vi "PID.vi"(0 "Numeric in":dbl, 1 "P_outer gain":dbl, 2 "Inner PID T/F":bool, 3 "Old (F), new (T) PID":bool, 4 "I_outer gain":dbl, 5 "D_outer gain":dbl, 6 "Velocity (Counts/interval)":i32, 7 "P_inner gain":dbl, 8 "Position (Counts)":i32, 9 "I_inner gain":dbl, 11 "D_inner gain":dbl) -> (14 "Numeric out":dbl)   [LabVIEW 2019]
uses:
  <vilib>/Simulation/Scripting/Companion Diagram/SimConfigNode/SimParams.ctl
  <vilib>/Simulation/Scripting/Companion Diagram/SimConfigNode/_simSolvers.ctl
  <vilib>/Simulation/Implementation/Shared/SIMSCR Execution Mode.ctl
  <vilib>/Simulation/Param Hierarchy/Typedefs/SIMPH Param Control Actions.ctl
  <vilib>/Simulation/Implementation/Shared/NILVSim_ParamChanged.vi
  <vilib>/Simulation/Implementation/Shared/NILVSIM_BeginStep.vi
  <vilib>/Simulation/Implementation/Shared/NILVSim_Manager.vi
  <vilib>/Utility/error.llb/Clear Errors.vi
  <vilib>/Simulation/Implementation/Shared/NILVSim_FinalizeModel.vi
  <vilib>/Simulation/Implementation/Shared/SIM Unbundle Sim Info.vi
  <vilib>/Simulation/Implementation/Shared/NILVSim_Initialize.vi
  <vilib>/Simulation/Utility/Implementation/NILVSim Get Time and IsAcceptedStep.vi
  <vilib>/Simulation/Implementation/Shared/SIMSH Read Queue.vi
  <vilib>/Simulation/Implementation/Shared/NILVSim_GetModelError.vi
  <vilib>/Simulation/Implementation/Shared/SIM Bundle Sim Info.vi
  <vilib>/Simulation/Implementation/XNodeFramework/SimXNode/SimX.xnode
  <vilib>/Simulation/Model Libraries/PID/SIM PID (Parallel).vi
  <vilib>/Simulation/Scripting/Companion Diagram/SimConfigNode/SimDog.xnode
  <vilib>/Simulation/Model Libraries/PID/SIM PID (Academic).vi
  <vilib>/ptbypt/NI_PtbyPt.lvlib
  <vilib>/Simulation/Implementation/Shared/NI_SIM_Implementation.lvlib
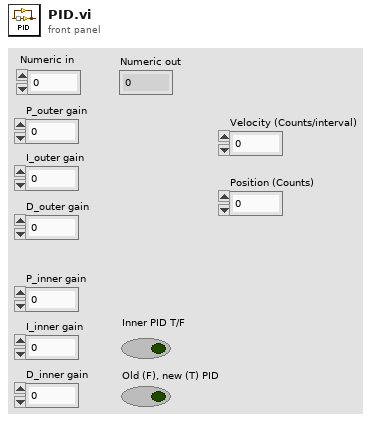
[diagram p1: front panel]
types:
  T1 = enum16{"Simulate to Completion", "Single Time-Step Simulation (Fixed Step Only)"}
  T2 = typedef "SIMSCR Execution Mode.ctl" = enum16{"Simulate to Completion", "Single Time-Step Simulation (Fixed Step Only)"}
  T3 = typedef "SIMPH Param Control Actions.ctl" = enum16{"get params", "set params"}
  T4 = cluster{"SIMSH Sim Time":dbl, "SIM PID Derivative Gain.vi":cluster{"output":dbl}, "SIM PID Derivative Gain.vi - SIMSH":cluster{"SIMSH Sim Time":dbl, "t 3":dbl, "Select 2":cluster{"s? t:f":dbl}, "Equal?":cluster{"x = y?":bool}, "Or":cluster{"x .or. y?":bool}, "Equal To 0?":cluster{"x = 0?":bool}}, "High Frequency [s] (Tf)":dbl, "Gain":cluster{"output":dbl}, "Summation":cluster{"Result":dbl}, "Integral Gain - series.vi":cluster{"output":dbl}, "Integral Gain - series.vi - SIMSH":cluster{"SIMSH Sim Time":dbl, "Select 2":cluster{"s? t:f":dbl}, "integral in gain?":bool, "Integrator":cluster{"output y(t)":dbl}, "Gain 2":cluster{"output":dbl}, "Select":cluster{"s? t:f":dbl}, "Equal To 0?":cluster{"x = 0?":bool}, "Reciprocal":cluster{"1/x":dbl}}}
  T5 = typedef "SimParams.ctl" = cluster{"Initial Time (s)":dbl, "Final Time (s)":dbl, "Step Size (s)":dbl, "ODE Solver":T6, "Minimum Step Size (s)":dbl, "Maximum Step Size (s)":dbl, "Relative Tolerance":dbl, "Absolute Tolerance":dbl, "Software Timing":bool, "Initial Step Size (s)":dbl, "Automatic Fixed Step Size?":bool, "Automatic Discrete Step Size?":bool, "Discrete Step Size (s)":dbl, "Calculate using Time Step":bool, "Solver Wired?":bool, "Prev.Frm.Expected End":u64, "Prev.Frm.Actual End":u64, "Prev.Frm.Finished Late?":bool, "Prev.Iter.Expected End":u64, "Prev.Iter.Actual End":u64, "Prev.Iter.Finished Late?":bool, "Expected Iteration Start":u64, "Actual Iteration Start":u64, "Expected Frame Start":u64, "Actual Frame Start":u64, "Source Name":string, "Name":string, "Period":i64, "Deadline":i64, "Offset":i64, "Start":i64, "Priority":i32, "Timeout":i32, "Processor":i32, "Mode":enum32{"No Change", "Process missed periods, maintain original phase", "Discard missed periods, maintain original phase", "Process missed periods, ignore original phase", "Discard missed periods, ignore original phase"}, "Wakeup reason":enum32{"Normal", "Aborted", "Asynchronous wakeup", "Timing source error", "Timed loop error", "Timeout"}, "Error":errorcluster, "Source Type":string, "Secondary Source Type":string, "Global End Time":u64, "Global Start Time":u64, "Full Solver Reset":bool, "Execution Mode":T2, "Nan/Inf Check":bool, "Custom Solver Library":string, "Solver Is Variable":bool, "custom solver name":string, "Signal Collection Decimation":u32}
  T6 = typedef "_simSolvers.ctl" = enum16{"Runge-Kutta 1 (Euler)", "Runge-Kutta 2", "Runge-Kutta 3", "Runge-Kutta 4", "Runge-Kutta 23 (variable)", "Runge-Kutta 45 (variable)", "BDF (variable)", "Adams-Moulton (variable)", "Rosenbrock (variable)", "Discrete States Only", "SDIRK 4 (variable)", "Radau 5 (variable)", "Radau 9 (variable)", "Radau 13 (variable)", "Radau [Variable Order] (variable)", "Gear's Method (variable)", "Linearizer", "State Query", "Trim Eval", "Custom Solver"}
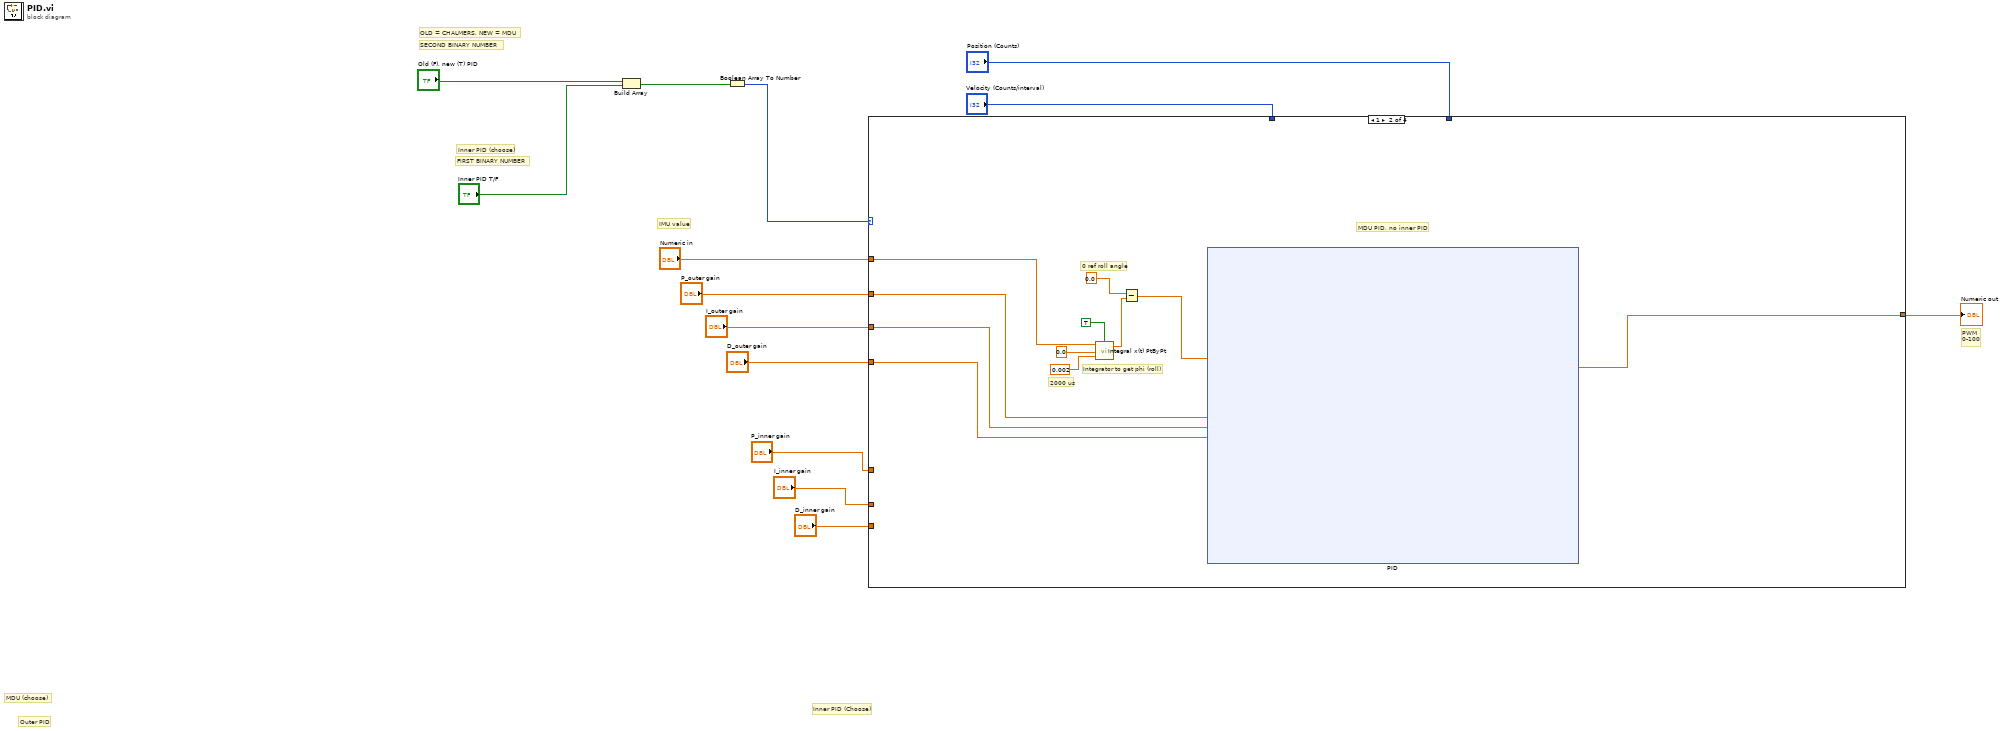
[diagram p0: block diagram]
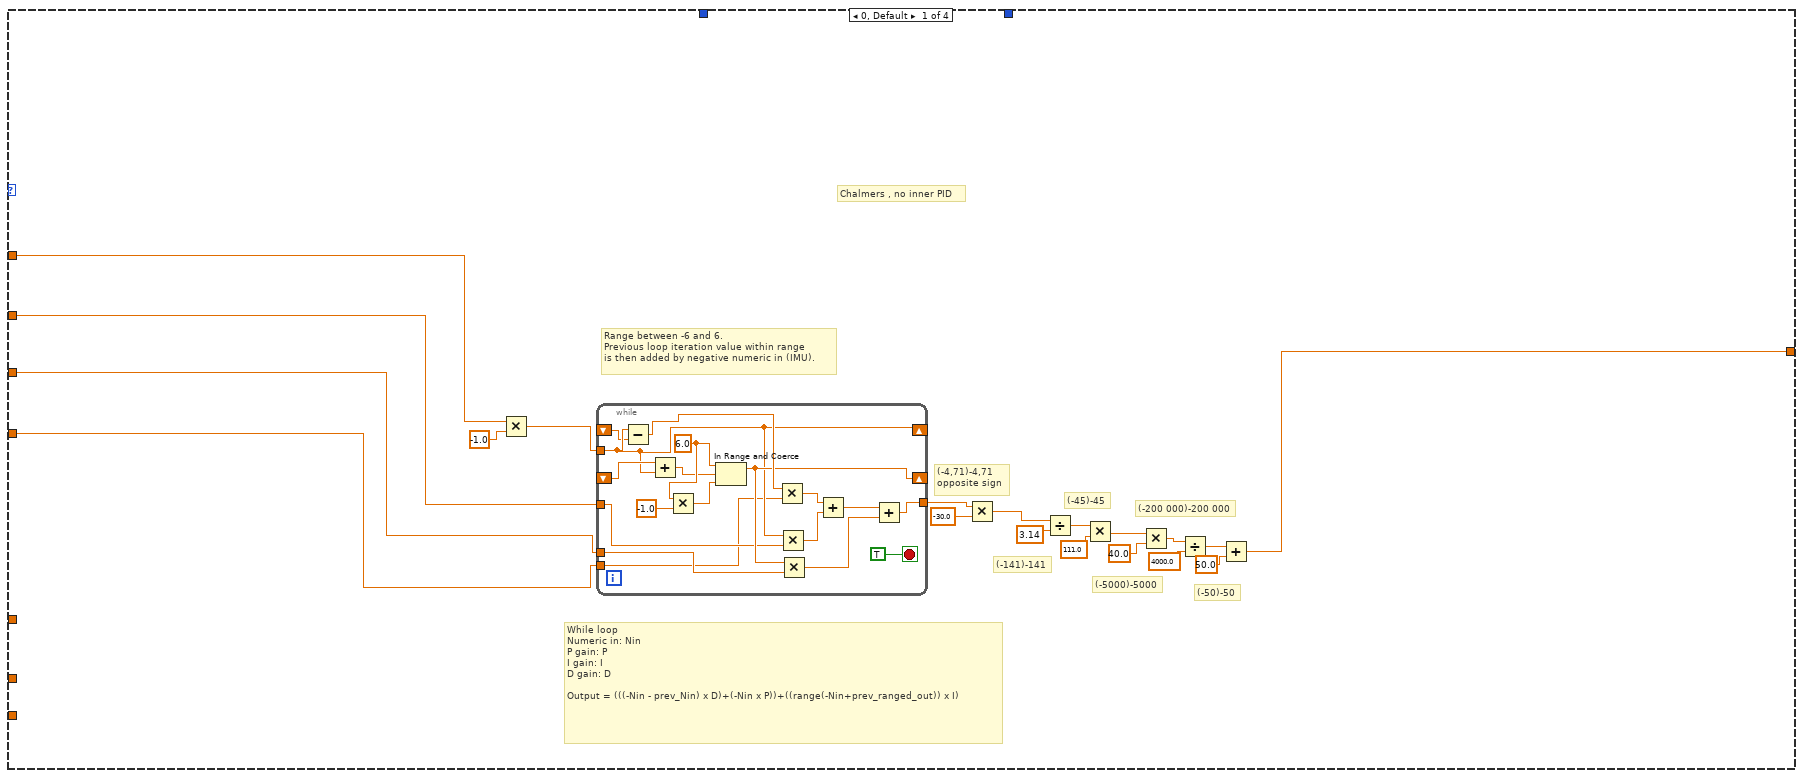
[diagram p2: hidden frame]
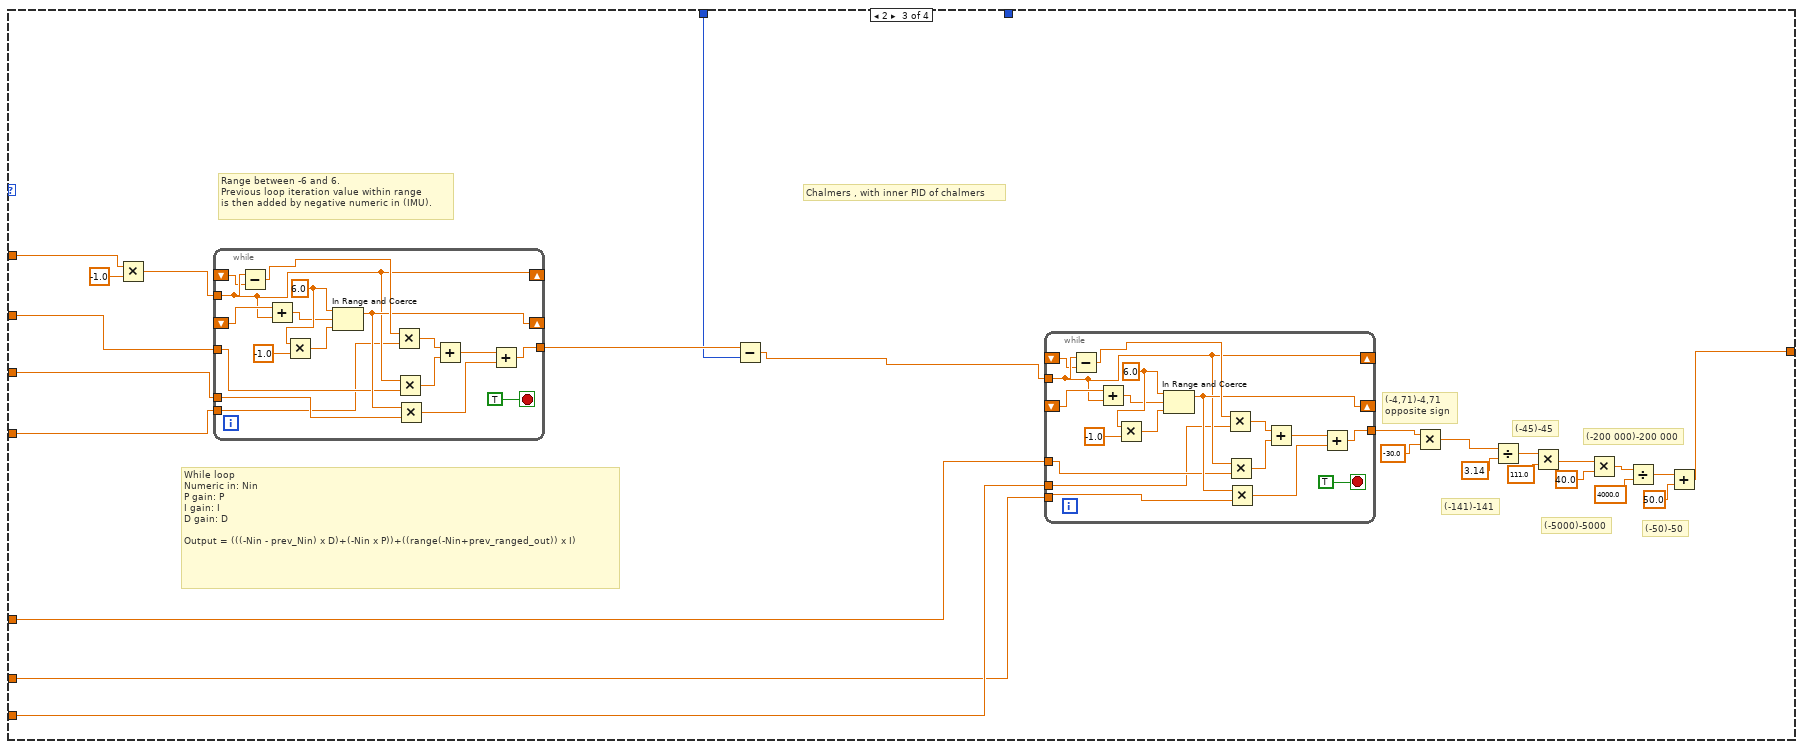
[diagram p3: hidden frame]
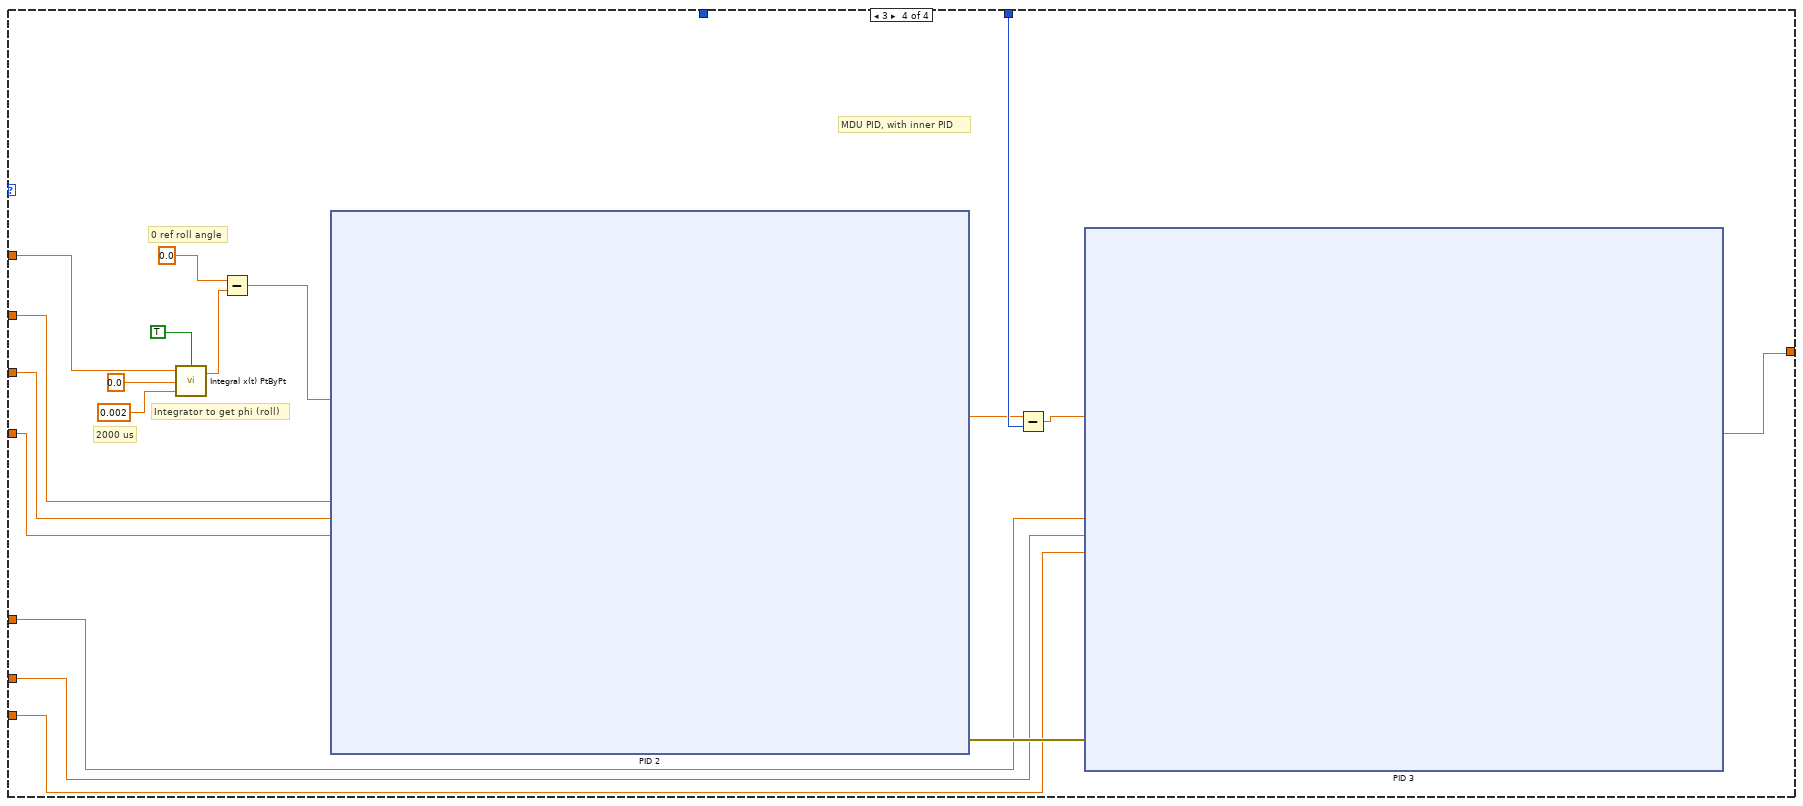
[diagram p4: hidden frame]
diagram:
  # "PWM\n0-100"
  # "OLD = CHALMERS, NEW = MDU"
  # "SECOND BINARY NUMBER"
  # "FIRST BINARY NUMBER"
  # "IMU value"
  # "Inner PID (Choose)"
  # "Outer PID"
  # "Inner PID (choose)"
  # "MDU (choose)"
  n1 = Build Array("Old (F), new (T) PID", "Inner PID T/F") -> (w4:bool[])
  n2 = Boolean Array To Number(Boolean array=w4) -> (number=w7:u64)
  n3 = case shown="1" w7 {
    tunnel: "P_inner gain" -> [_ _ w322 w375]
    tunnel: "D_inner gain" -> [_ _ w321 w373]
    tunnel: "I_inner gain" -> [_ _ w320 w374]
    tunnel: "D_outer gain" -> [w16 w52 w318 w378]
    tunnel: "I_outer gain" -> [w17 w53 w317 w379]
    tunnel: "P_outer gain" -> [w18 w54 w316 w380]
    tunnel: "Numeric in" -> [w19 w59 w315 w383]
    tunnel: "Velocity (Counts/interval)" -> [_ _ w311 _]
    tunnel: [w15 w55 w310 w372] -> w3
    tunnel: "Position (Counts)" -> [_ _ _ w382]
    frame 0, Default {
      # "Chalmers , no inner PID"
      # "Range between -6 and 6.\nPrevious loop iteration value within range\nis then added by negative numeric in (IMU)."
      # "While loop\nNumeric in: Nin\nP gain: P\nI gain: I\nD gain: D\n\nOutput = (((-Nin - prev_Nin) x D)+(-Nin x P))+((range(-Nin+prev_ranged_out)) x I)"
      # "(-4,71)-4,71\nopposite sign"
      # "(-141)-141"
      # "(-45)-45"
      # "(-5000)-5000"
      # "(-200 000)-200 000"
      # "(-50)-50"
      n4 = Multiply(x=w19, y=-1.0) -> (x*y=w20:dbl)
      n5 = while {
        shift-right: [w44] -> _
        shift-left: _ -> [w50]
        tunnel: w20 -> [w38]
        shift-right: [w38] -> _
        shift-left: _ -> [w37]
        tunnel: w18 -> [w36]
        tunnel: w17 -> [w35]
        tunnel: w16 -> [w34]
        tunnel: [w39] -> w28
        stop <- TRUE stop-if-true
        w47 = 6.0 ("upper limit")
        n6 = Subtract(x=w38, y=w37) -> (x-y=w45:dbl)
        n7 = Add(x=w50, y=w38) -> (x+y=w46:dbl)
        n8 = Multiply(x=w47, y=-1.0) -> (x*y=w48:dbl)
        n9 = In Range and Coerce(upper limit=w47, x=w46, lower limit=w48) -> (coerced(x)=w44:dbl)  [unwired: 1 out]
        n10 = Multiply(x=w45, y=w34) -> (x*y=w43:dbl)
        n11 = Multiply(x=w38, y=w36) -> (x*y=w42:dbl)
        n12 = Multiply(x=w44, y=w35) -> (x*y=w40:dbl)
        n13 = Add(x=w43, y=w42) -> (x+y=w41:dbl)
        n14 = Add(x=w41, y=w40) -> (x+y=w39:dbl)
      }
      n15 = Multiply(x=w28, y=-30.0) -> (x*y=w29:dbl)
      n16 = Divide(x=w29, y=3.14) -> (x/y=w30:dbl)
      n17 = Multiply(x=w30, y=111.0) -> (x*y=w31:dbl)
      n18 = Multiply(x=w31, y=40.0) -> (x*y=w32:dbl)
      n19 = Divide(x=w32, y=4000.0) -> (x/y=w33:dbl)
      n20 = Add(x=w33, y=50.0) -> (x+y=w15:dbl)
    }
    frame 1 {
      # "Integrator to get phi (roll)"
      # "2000 us"
      # "0 ref roll angle"
      # "MDU PID, no inner PID"
      n21 = call <vilib>:"Integral x(t) PtByPt.vi"("initialize"=TRUE, "dt"=0.002, "initial condition"=0.0, "x"=w59) -> ("integral x(t)"=w56:dbl)  [unwired: 1 out]
      n22 = Subtract(x=0.0, y=w56) -> (x-y=w61:dbl)
      n23 = xnode "PID"("Error"=w61, "Proportional Gain"=w54, "Integral Gain"=w53, "Derivative Gain"=w52) -> ("Output"=w55:dbl)  [unwired: 2 in, 11 out]
    }
    frame 2 {
      # "Chalmers , with inner PID of chalmers"
      # "Range between -6 and 6.\nPrevious loop iteration value within range\nis then added by negative numeric in (IMU)."
      # "While loop\nNumeric in: Nin\nP gain: P\nI gain: I\nD gain: D\n\nOutput = (((-Nin - prev_Nin) x D)+(-Nin x P))+((range(-Nin+prev_ranged_out)) x I)"
      # "(-4,71)-4,71\nopposite sign"
      # "(-141)-141"
      # "(-45)-45"
      # "(-5000)-5000"
      # "(-200 000)-200 000"
      # "(-50)-50"
      n24 = Multiply(x=w315, y=-1.0) -> (x*y=w314:dbl)
      n25 = while {
        shift-right: [w345] -> _
        shift-left: _ -> [w351]
        tunnel: w314 -> [w339]
        shift-right: [w339] -> _
        shift-left: _ -> [w338]
        tunnel: w316 -> [w337]
        tunnel: w317 -> [w336]
        tunnel: w318 -> [w335]
        tunnel: [w340] -> w312
        stop <- TRUE stop-if-true
        w348 = 6.0 ("upper limit")
        n26 = Subtract(x=w339, y=w338) -> (x-y=w346:dbl)
        n27 = Add(x=w351, y=w339) -> (x+y=w347:dbl)
        n28 = Multiply(x=w348, y=-1.0) -> (x*y=w349:dbl)
        n29 = In Range and Coerce(upper limit=w348, x=w347, lower limit=w349) -> (coerced(x)=w345:dbl)  [unwired: 1 out]
        n30 = Multiply(x=w346, y=w335) -> (x*y=w344:dbl)
        n31 = Multiply(x=w339, y=w337) -> (x*y=w343:dbl)
        n32 = Multiply(x=w345, y=w336) -> (x*y=w341:dbl)
        n33 = Add(x=w344, y=w343) -> (x+y=w342:dbl)
        n34 = Add(x=w342, y=w341) -> (x+y=w340:dbl)
      }
      n35 = Subtract(x=w312, y=w311) -> (x-y=w313:dbl)
      n36 = while {
        shift-right: [w363] -> _
        shift-left: _ -> [w369]
        tunnel: w313 -> [w357]
        shift-right: [w357] -> _
        shift-left: _ -> [w356]
        tunnel: w322 -> [w355]
        tunnel: w321 -> [w354]
        tunnel: [w358] -> w329
        tunnel: w320 -> [w353]
        stop <- TRUE stop-if-true
        w366 = 6.0 ("upper limit")
        n37 = Subtract(x=w357, y=w356) -> (x-y=w364:dbl)
        n38 = Add(x=w369, y=w357) -> (x+y=w365:dbl)
        n39 = Multiply(x=w366, y=-1.0) -> (x*y=w367:dbl)
        n40 = In Range and Coerce(upper limit=w366, x=w365, lower limit=w367) -> (coerced(x)=w363:dbl)  [unwired: 1 out]
        n41 = Multiply(x=w364, y=w354) -> (x*y=w362:dbl)
        n42 = Multiply(x=w357, y=w355) -> (x*y=w361:dbl)
        n43 = Multiply(x=w363, y=w353) -> (x*y=w359:dbl)
        n44 = Add(x=w362, y=w361) -> (x+y=w360:dbl)
        n45 = Add(x=w360, y=w359) -> (x+y=w358:dbl)
      }
      n46 = Multiply(x=w329, y=-30.0) -> (x*y=w330:dbl)
      n47 = Divide(x=w330, y=3.14) -> (x/y=w331:dbl)
      n48 = Multiply(x=w331, y=111.0) -> (x*y=w332:dbl)
      n49 = Multiply(x=w332, y=40.0) -> (x*y=w333:dbl)
      n50 = Divide(x=w333, y=4000.0) -> (x/y=w334:dbl)
      n51 = Add(x=w334, y=50.0) -> (x+y=w310:dbl)
    }
    frame 3 {
      # "Integrator to get phi (roll)"
      # "2000 us"
      # "0 ref roll angle"
      # "MDU PID, with inner PID"
      n52 = call <vilib>:"Integral x(t) PtByPt.vi"("initialize"=TRUE, "dt"=0.002, "initial condition"=0.0, "x"=w383) -> ("integral x(t)"=w384:dbl)  [unwired: 1 out]
      n53 = Subtract(x=0.0, y=w384) -> (x-y=w381:dbl)
      n54 = xnode "PID 2"("Error"=w381, "Proportional Gain"=w380, "Integral Gain"=w379, "Derivative Gain"=w378) -> ("Output"=w377:dbl, "error out"=w376:errorcluster)  [unwired: 2 in, 10 out]
      n55 = Subtract(x=w377, y=w382) -> (x-y=w371:dbl)
      n56 = xnode "PID 3"("Error"=w371, "Proportional Gain"=w375, "Integral Gain"=w374, "Derivative Gain"=w373, "error in"=w376) -> ("Output"=w372:dbl)  [unwired: 1 in, 11 out]
    }
  }
  "Numeric out" <- w3
